vi "2d queue.vi"() -> ()   [LabVIEW 2023]
uses:
  control/Data Form.ctl
  control/file structure.ctl
  <vilib>/Analysis/1siggen.llb/Ramp Pattern by Samples.vi
  queue/Front Panel Message Queue.lvlib
  <vilib>/Analysis/NI_AALBase.lvlib
panel:
  in  "data value reference":refnum<data-value>
  out "XY Graph":cluster{"Ramp Pattern":dbl[], i32[]}(graph)
  out "Data Form":T1
  out "error out":errorcluster
  in  "error in":errorcluster
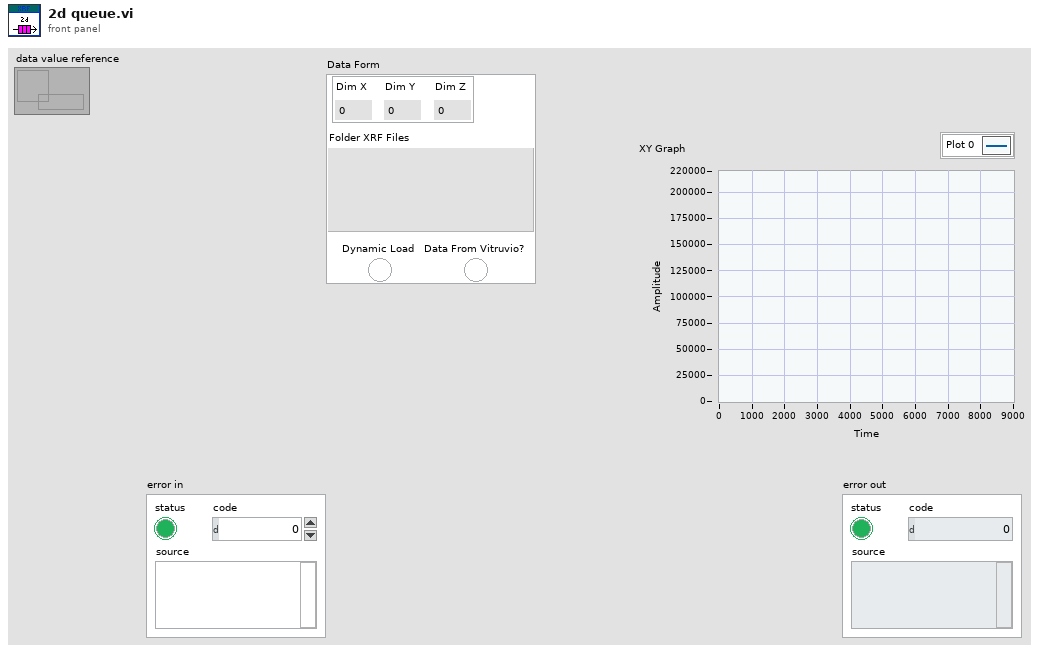
[diagram p1: front panel]
types:
  T1 = typedef "Data Form.ctl" = cluster{"Dimensions":cluster{"Dim X":i32, "Dim Y":i32, "Dim Z":i32}, "Folder XRF Files":path, "Dynamic Load":bool, "Data From Vitruvio?":bool}
  T2 = typedef "Front Panel Message Queue.lvlib/2d3d Message Queues.ctl" = cluster{"Main":refnum<queue>, "2d":refnum<queue>, "3d":refnum<queue>}
  T3 = typedef "file structure.ctl" = cluster{"Colonna":i32, "Offset Righe":i32, "Coda Righe":i32, "Transpose":bool}
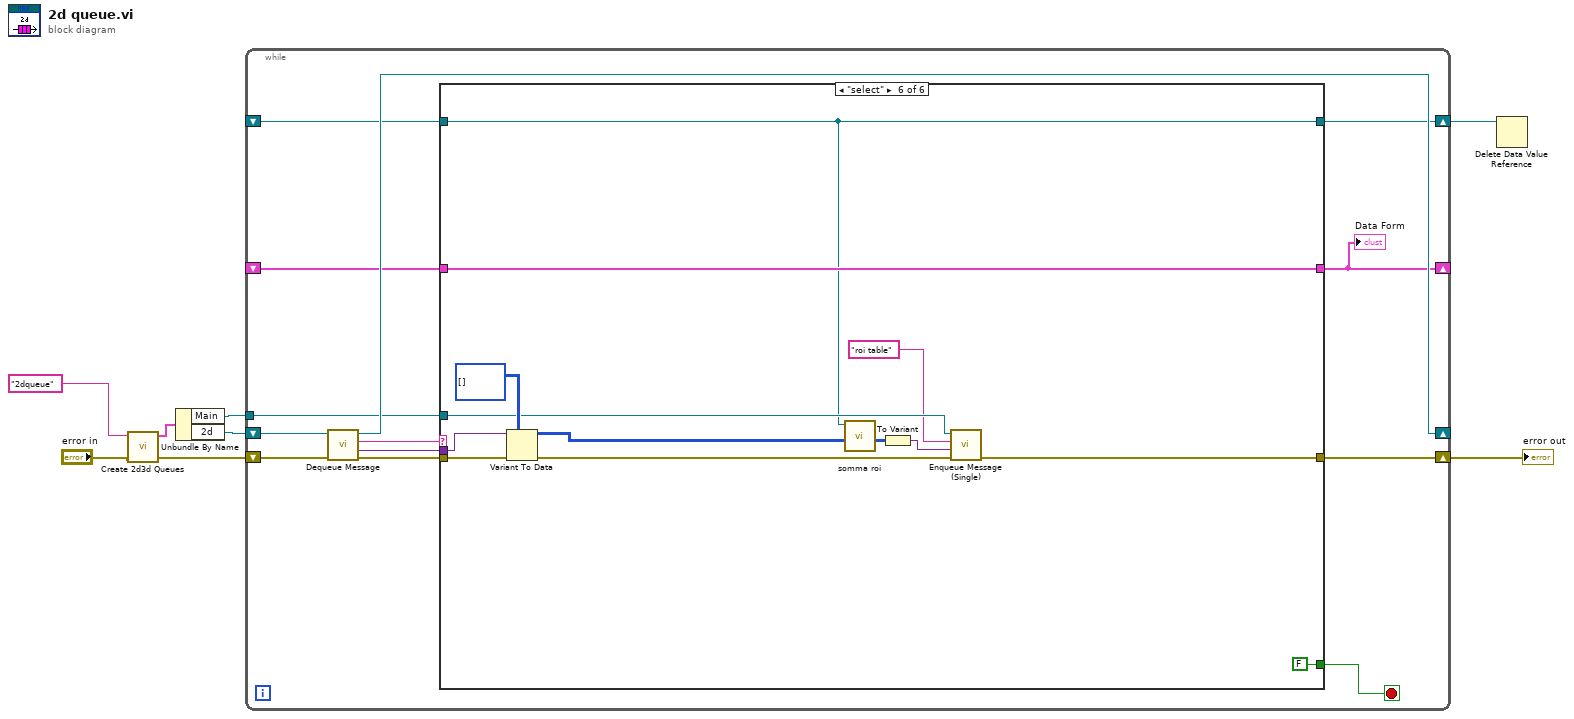
[diagram p0: block diagram]
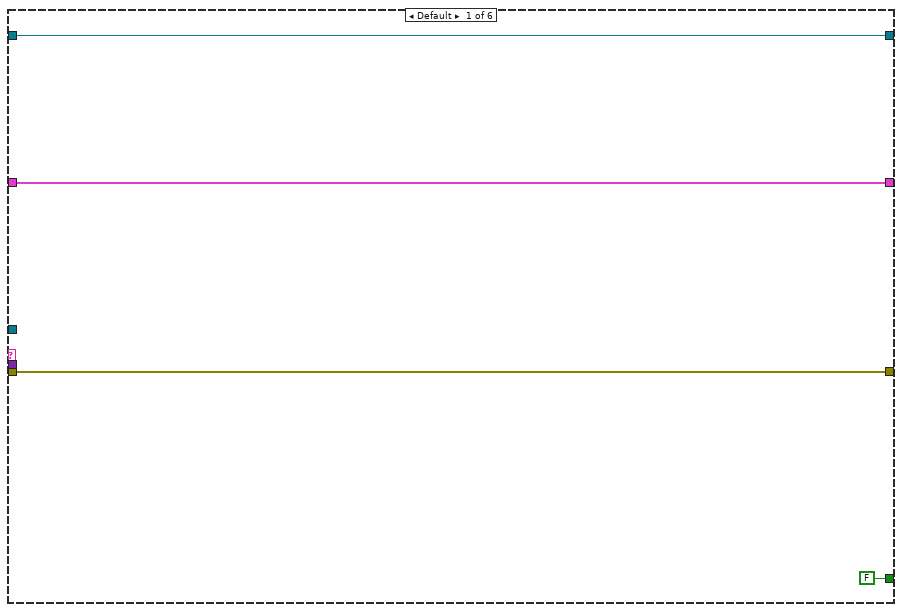
[diagram p2: hidden frame]
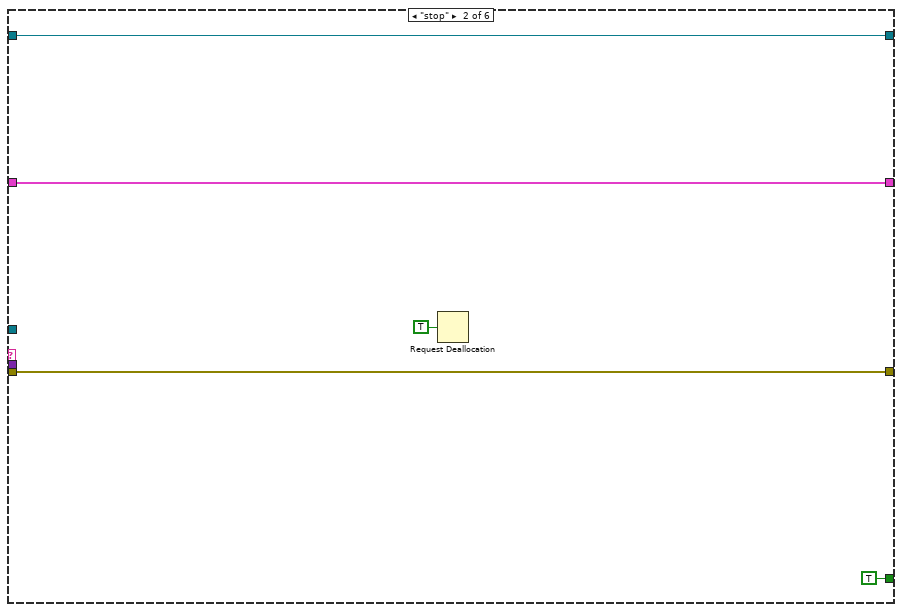
[diagram p3: hidden frame]
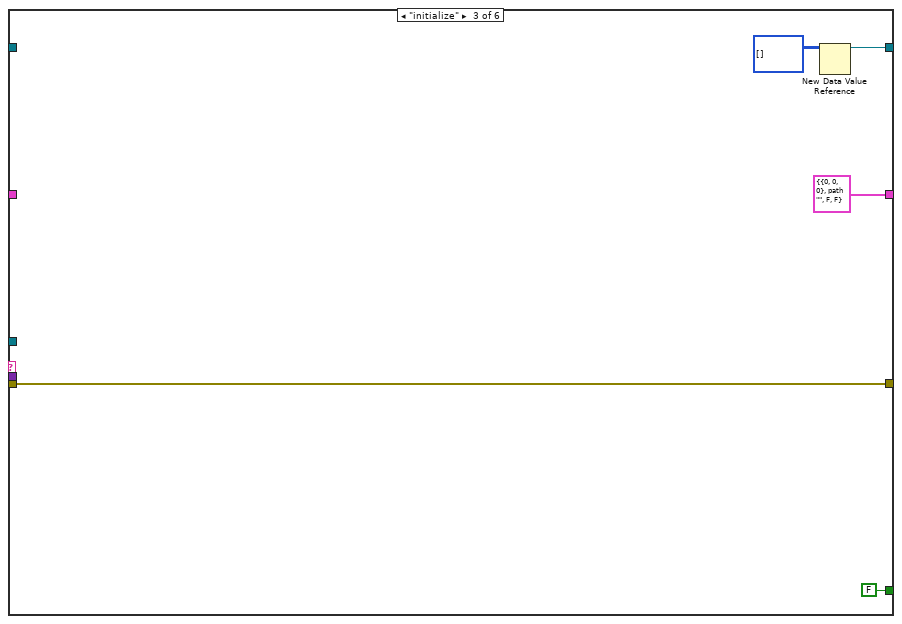
[diagram p4: hidden frame]
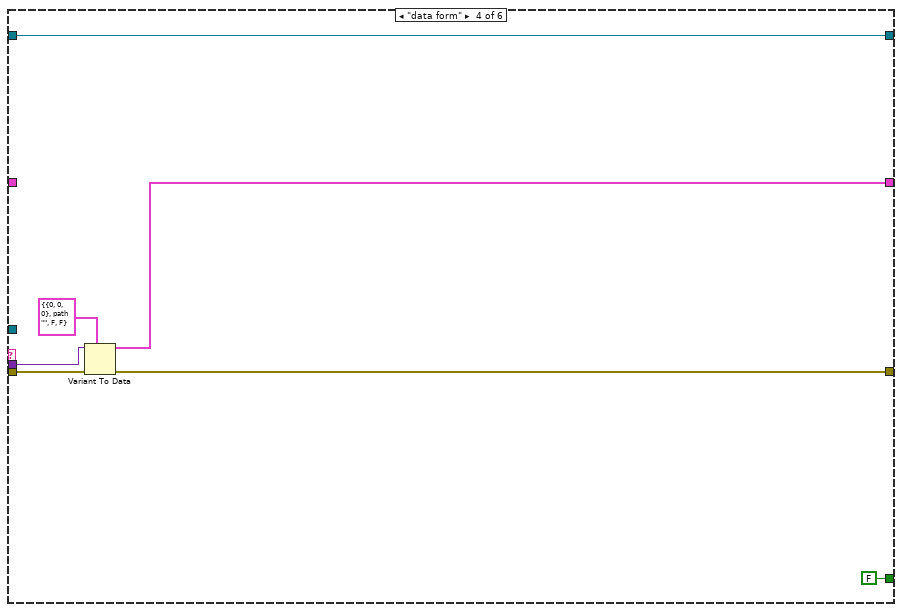
[diagram p5: hidden frame]
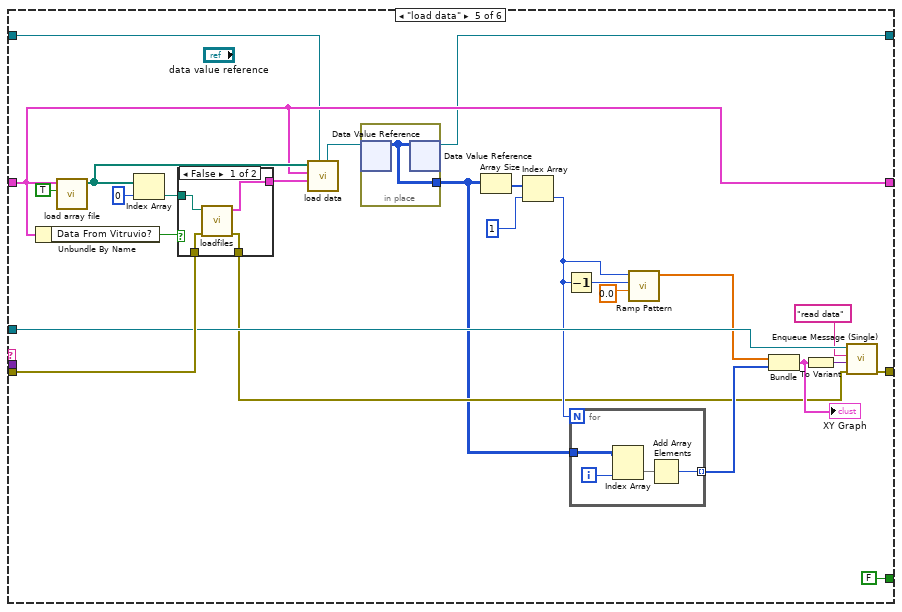
[diagram p6: hidden frame]
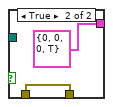
[diagram p7: hidden frame]
diagram:
  n1 = call "Create 2d3d Queues.vi"("error in (no error)"="error in", "name"="2dqueue") -> ("error out"=w5:errorcluster, "Message Queues"=w3:T2)  [unwired: 8 in]
  n2 = Unbundle By Name(w3) -> ("Main"=w2:refnum<queue>, "2d"=w8:refnum<queue>)
  n3 = while {
    shift-right: [w18] -> _
    shift-left: w8 -> [w20]
    shift-right: [w15] -> w7
    shift-left: w5 -> [w21]
    shift-right: [w12] -> _
    shift-left: _ -> [w13]
    tunnel: w2 -> [w11]
    shift-right: [w10] -> w1
    shift-left: _ -> [w9]
    stop <- w16 stop-if-true
    n4 = call "Dequeue Message.vi"("error in (no error)"=w21, "Message Queue"=w20) -> ("error out"=w19:errorcluster, "Message Data"=w14:variant, "Message"=w17:string, "dup Message Queue"=w18:refnum<queue>)  [unwired: 5 in, 1 out]
    n5 = case shown="\"select\"" w17 {
      tunnel: w19 -> [w24 w29 w31 w42 w64 w91]
      tunnel: [FALSE TRUE FALSE FALSE FALSE FALSE] -> w16
      tunnel: [w24 w29 w31 w38 w59 w83] -> w15
      tunnel: w14 -> [_ _ _ w41 _ w90]
      tunnel: [w23 w28 T1 {"Dimensions"={"Dim X"=0, "Dim Y"=0, "Dim Z"=0}, "Folder XRF Files"=path "", "Dynamic Load"=FALSE, "Data From Vitruvio?"=FALSE} ("Data Form") w39 w55 w82] -> w12
      tunnel: w13 -> [w23 w28 _ _ w55 w82]
      tunnel: w11 -> [_ _ _ _ w58 w85]
      tunnel: [w22 w26 w32 w36 w44 w80] -> w10
      tunnel: w9 -> [w22 w26 _ w36 w46 w80]
      frame Default {
      }
      frame "stop" {
        n6 = Request Deallocation(TRUE ("flag")) -> ()
      }
      frame "initialize" {
        n7 = New Data Value Reference(data value=i32[][] [] ("Data Loaded")) -> (data value reference=w32:refnum<data-value>)  [unwired: 1 in, 1 out]
      }
      frame "data form" {
        n8 = Variant To Data(error in=w42, type=T1 {"Dimensions"={"Dim X"=0, "Dim Y"=0, "Dim Z"=0}, "Folder XRF Files"=path "", "Dynamic Load"=FALSE, "Data From Vitruvio?"=FALSE} ("Data Form"), Variant=w41) -> (data=w39:T1, error out=w38:errorcluster)
      }
      frame "load data" {
        n9 = Unbundle By Name(w55) -> ("Data From Vitruvio?"=w54:bool)
        n10 = call "load array file.vi"("2d?"=TRUE, "Data Form"=w55) -> ("File Array Out"=w63:path[])  [unwired: 9 in]
        n11 = Index Array(array=w63, index=0) -> (element=w65:path)
        n12 = case shown="False" w54 {
          tunnel: w65 -> [w71 _]
          tunnel: w64 -> [w73 w75]
          tunnel: [w70 T3 {"Colonna"=0, "Offset Righe"=0, "Coda Righe"=0, "Transpose"=TRUE} ("File Structure")] -> w62
          tunnel: [w72 w75] -> w47
          frame False {
            n13 = call "loadfiles.vi"("Error In"=w73, "First Spectrum"=w71) -> ("Error Out"=w72:errorcluster, "File Structure"=w70:T3)  [unwired: 8 in]
          }
          frame True {
          }
        }
        n14 = call "load data.vi"("Data loaded reference In"=w46, "File Structure"=w62, "Data Form"=w55, "File Array In"=w63) -> ("Data loaded reference Out"=w45:refnum<data-value>)  [unwired: 7 in]
        n15 = in-place {
          in-place-border: [w69] -> w43
          n16 = in-place-dvr #1(w45) -> (w69:i32[][])  [unwired: 1 out]
          n17 = in-place-dvr #1(w69) -> (w44:refnum<data-value>)  [unwired: 1 out]
        }
        n18 = Array Size(array=w43) -> (size(s)=w61:i32[])
        n19 = Index Array(array=w61, index=1) -> (element=w51:i32)
        n20 = Decrement(x=w51) -> (x-1=w53:i32)
        n21 = for {
          N: w51 -> [_]
          tunnel: w43 -> [w78]
          tunnel: [w76] -> w49 mode=indexing
          i -> [w77]
          n22 = Index Array(array=w78, index (col)=w77) -> (element=w79:i32[])  [unwired: 1 in]
          n23 = Add Array Elements(numeric array=w79) -> (sum=w76:i32)
        }
        n24 = call-poly <vilib>:"Ramp Pattern.vi"("start"=0.0, "end"=w53, "samples"=w51) -> ("Ramp Pattern"=w50:dbl[])  [unwired: 7 in, 1 out]
        n25 = Bundle("Ramp Pattern"=w50, w49) -> (w48:cluster{"Ramp Pattern":dbl[], i32[]})  [unwired: 1 in]
        "XY Graph" <- w48
        n26 = To Variant(anything=w48) -> (Variant=w56:variant)
        n27 = call "Enqueue Message (Single).vi"("error in (no error)"=w47, "Message Data"=w56, "Message"="read data", "Message Queue"=w58) -> ("error out"=w59:errorcluster)  [unwired: 6 in, 1 out]
      }
      frame "select" {
        n28 = Variant To Data(error in=w91, type=i32[][] [] ("ROIs Min Max"), Variant=w90) -> (data=w88:i32[][], error out=w81:errorcluster)
        n29 = call "somma roi.vi"("ROIs Min Max"=w88, "Data loaded reference In"=w80) -> ("ROIs Array Out"=w87:i32[][])  [unwired: 9 in]
        n30 = To Variant(anything=w87) -> (Variant=w86:variant)
        n31 = call "Enqueue Message (Single).vi"("error in (no error)"=w81, "Message Data"=w86, "Message"="roi table", "Message Queue"=w85) -> ("error out"=w83:errorcluster)  [unwired: 6 in, 1 out]
      }
    }
    "Data Form" <- w12
  }
  "error out" <- w7
  n32 = Delete Data Value Reference(data value reference=w1) -> ()  [unwired: 1 in, 2 out]
